vi "OEE_MAIN.vi"() -> ()   [LabVIEW 2020]
uses:
  OEE/FGV/SQL_raw_data/OEE_SQL_raw_data.ctl
  OEE/ini/typedef/OEE_all_config_info.ctl
  OEE/ini/typedef/OEE_main_ini_file.ctl
  OEE/queues/typedef/OEE_queue_refnums.ctl
  OEE/queues/typedef/OEE_MAIN_queue_element.ctl
  OEE/MAIN/OEE_MAIN_sequence_state.ctl
  OEE/queues/typedef/OEE_SCREEN_1_queue_element.ctl
  OEE/SCREEN_1/OEE_SCREEN_1_sequence_state.ctl
  OEE/queues/typedef/OEE_SCREEN_2_queue_element.ctl
  OEE/SCREEN_2/OEE_SCREEN_2_sequence_state.ctl
  OEE/queues/typedef/OEE_PULSE_queue_element.ctl
  OEE/PULSE/OEE_PULSE_sequence_state.ctl
  OEE/queues/typedef/OEE_GRAPH_TOGGLE_TIMER_queue_element.ctl
  OEE/SCREEN_2/GRAPH_TOGGLE_TIMER/OEE_GRAPH_TOGGLE_TIMER_sequence_state.ctl
  OEE/FGV/SQL_connection/FGV_OEE_SQL_connection.ctl
  OEE/FGV/SQL_raw_data/FGV_OEE_SQL_raw_data.ctl
  OEE/FGV/reference_selector/FGV_OEE_reference_selector.ctl
  OEE/FGV/reference_selector/OEE_reference_selecotr_references.ctl
  _misc/AULocalize/SubVIs/RegisterVI.vi
  _misc/AULocalize/SubVIs/Get Localized Phrase Compact Interface 0D.vi
panel:
  out "language_header":string caption="ЯЗЫК"
  out "status_info_header":string caption="ИНФОРМАЦИЯ О СТАТУСЕ"
  out "reference_selector_header":string caption="ТИП ДЕТАЛИ"
  out "time_source_header":string caption="TIME SOURCE"
  in  "language_russian":bool
  in  "language_english":bool
  in  "time_selector_btn":bool
  in  "time_selector":timestamp format="%<%x %H:%M:%S>T"
  in  "time_source_selector":enum32{"system_time", "manual_time"}(radio)
  in  "reload_reference_list":bool
  in  "reference_selector":u16(ring) items=["REF_1", "REF_2"]
  out "SQL_raw_data_out":T1
  out "update_pulse":bool=TRUE caption="Update Pulse:"
  in  "toggle_pulses":bool
  out "SQL_connection_status":bool=TRUE caption="SQL Connection Status:"
  in  "STOP":bool
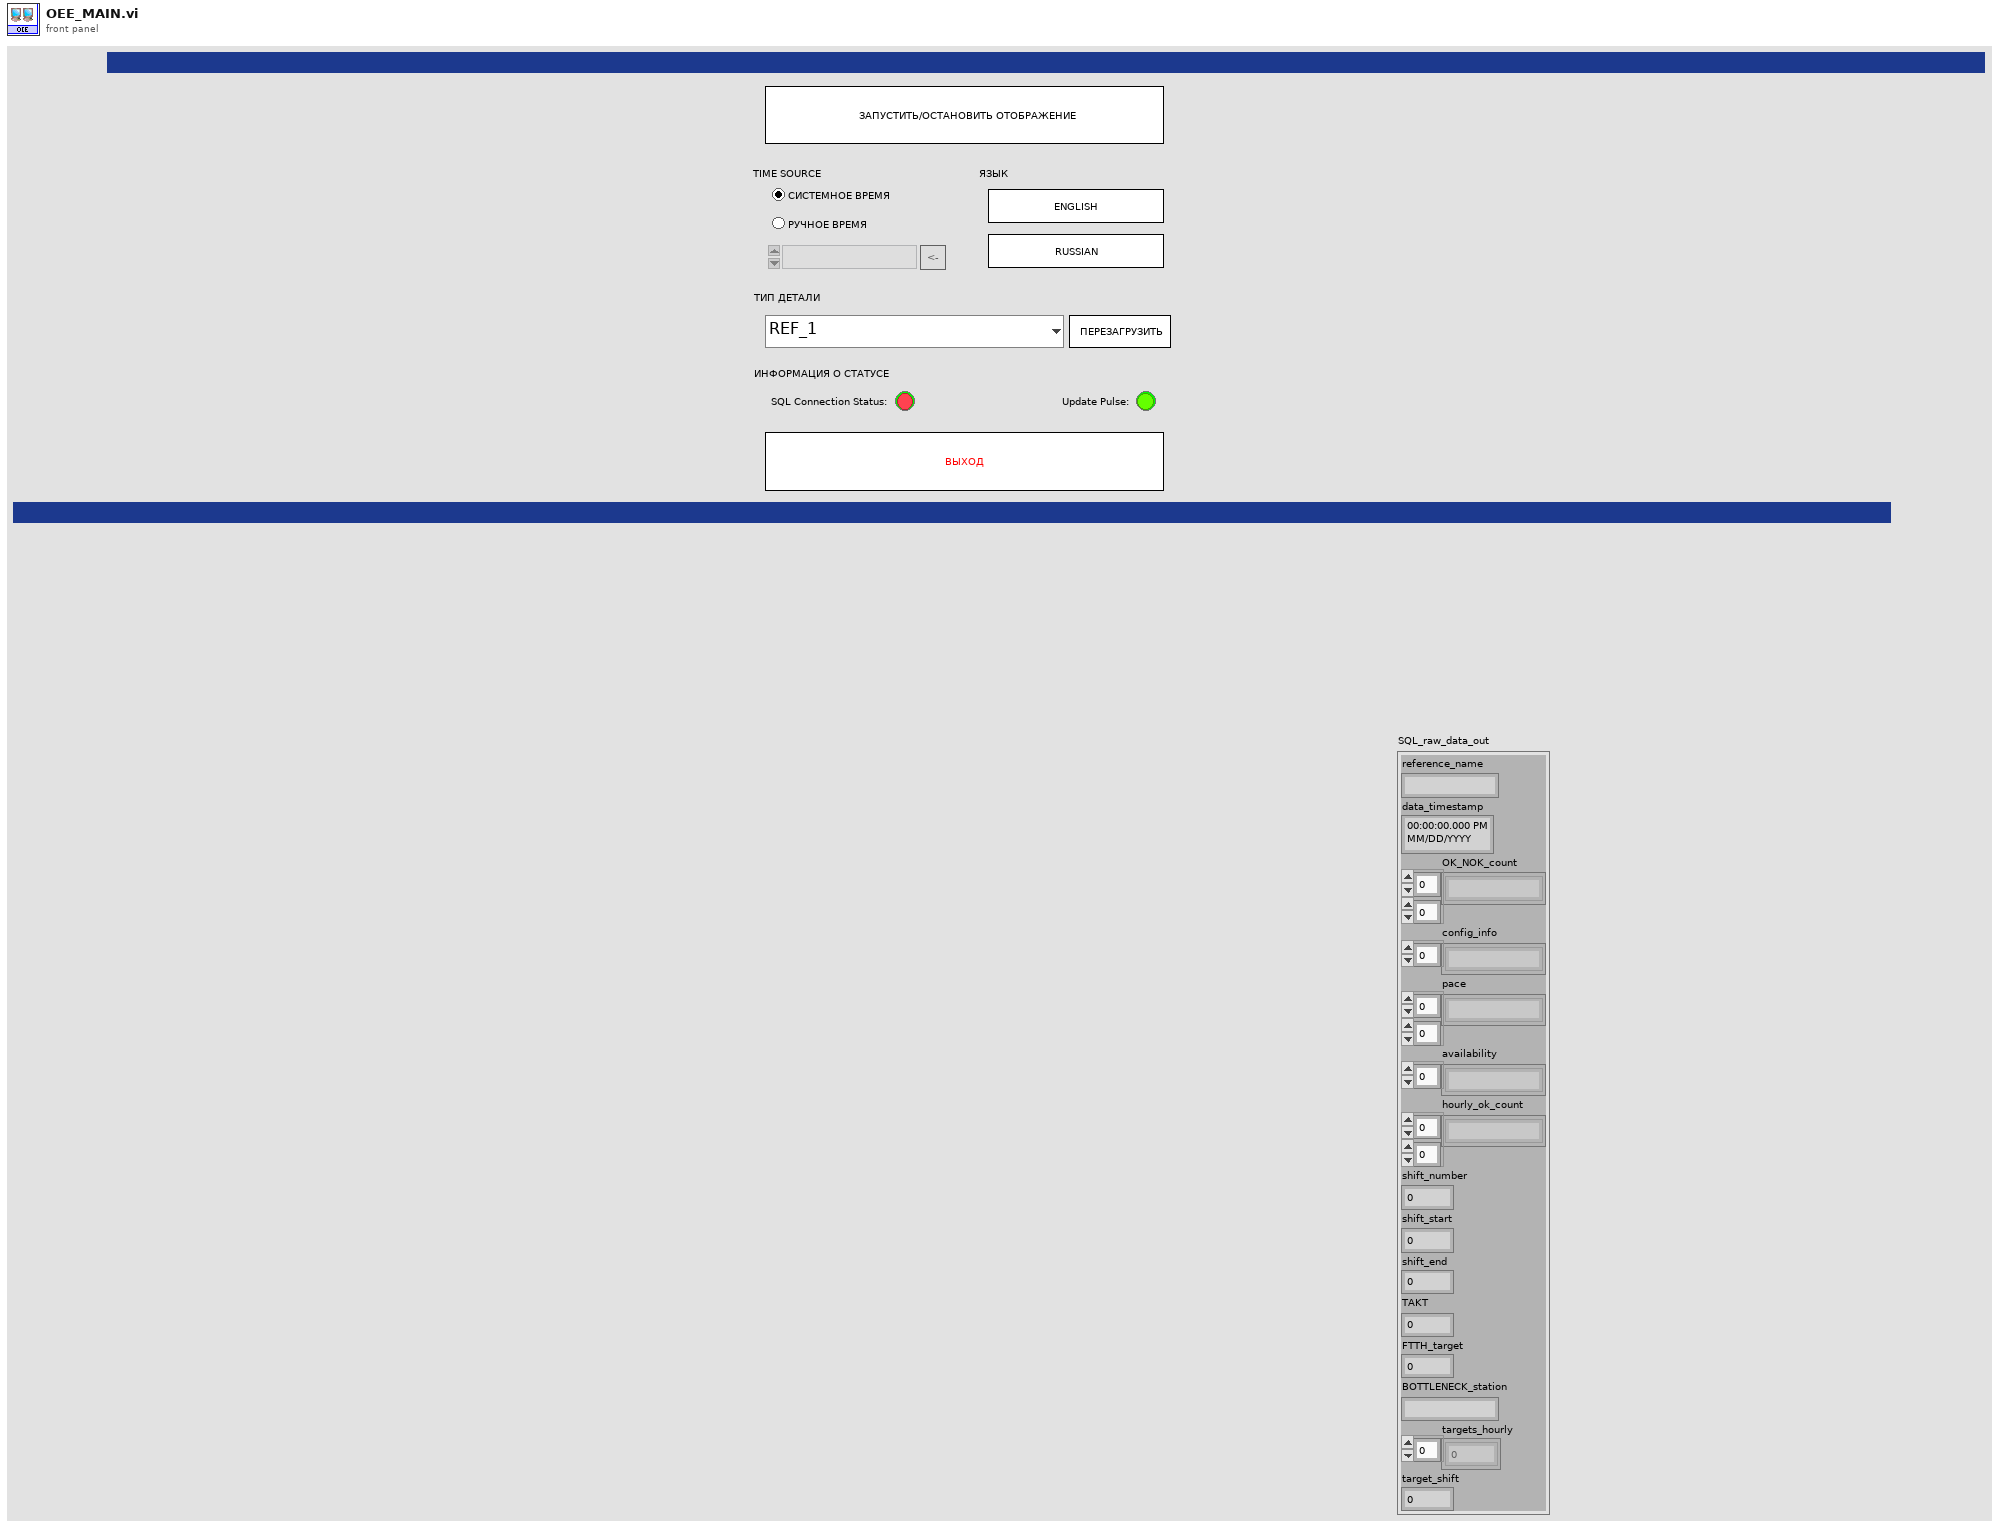
[diagram p1: front panel]
types:
  T1 = typedef "OEE_SQL_raw_data.ctl" = cluster{"reference_name":string, "data_timestamp":timestamp, "OK_NOK_count":string[][], "config_info":string[], "pace":string[][], "availability":string[], "hourly_ok_count":string[][], "shift_number":i8, "shift_start":i8, "shift_end":i8, "TAKT":u16, "FTTH_target":u16, "BOTTLENECK_station":string, "targets_hourly":u16[], "target_shift":u16}
  T2 = typedef "OEE_reference_selecotr_references.ctl" = cluster{"reference_list":string[], "reference_selector":refnum<vi>, "reload_reference_list":refnum<vi>, "toggle_pulses":refnum<vi>}
  T3 = typedef "FGV_OEE_reference_selector.ctl" = enum16{"initialize", "set_values", "enable", "disable", "disable_gray", "get_reference_list", "get_active_reference"}
  T4 = typedef "FGV_OEE_SQL_raw_data.ctl" = enum16{"initialize", "set_reference_name", "set_timestamp", "set_OK_NOK_count", "set_config_info", "set_pace", "set_availability", "set_hourly_ok_count", "set_targets", "get_all_info"}
  T5 = typedef "FGV_OEE_SQL_connection.ctl" = enum16{"initialize", "connect", "read_tables", "read_columns", "SELECT", "INSERT", "UPDATE", "DELETE", "EXEC + headers", "EXEC", "TRANSACTION", "connection_active?", "disconnect"}
  T6 = typedef "OEE_all_config_info.ctl" = cluster{"main_ini_file":T7, "SQL Password":string, "queue_refnums":T8}
  T7 = typedef "OEE_main_ini_file.ctl" = cluster{"SQL Driver":string, "SQL Server":string, "SQL Database":string, "SQL UID":string, "Reference table":string, "Reference history":string, "Archivisation CFG table":string, "Archivisation CFG history":string, "User table":string, "User history":string, "Default reference":string, "Update pulse[ms]":i32, "default language":string, "SCREEN 1 Left":i16, "SCREEN 1 Top":i16, "SCREEN 1 Width":i16, "SCREEN 1 Height":i16, "SCREEN 2 Left":i16, "SCREEN 2 Top":i16, "SCREEN 2 Width":i16, "SCREEN 2 Height":i16}
  T8 = typedef "OEE_queue_refnums.ctl" = cluster{"MAIN_queue":refnum<queue>, "SCREEN_1_queue":refnum<queue>, "SCREEN_2_queue":refnum<queue>, "PULSE_queue":refnum<queue>, "GRAPH_TOGGLE_queue":refnum<queue>}
  T9 = typedef "OEE_MAIN_sequence_state.ctl" = enum16{"initialize", "get_next_state", "get_SQL_data", "update_displays", "error", "stop"}
  T10 = typedef "OEE_PULSE_sequence_state.ctl" = enum16{"initialize", "get_next_state", "start_pulses", "stop_pulses", "pulse", "error", "stop"}
  T11 = typedef "OEE_GRAPH_TOGGLE_TIMER_queue_element.ctl" = cluster{"state":T12, "variable":variant}
  T12 = typedef "OEE_GRAPH_TOGGLE_TIMER_sequence_state.ctl" = enum16{"initialize", "get_next_state", "start_toggling", "stop_toggling", "do_toggle", "error", "stop"}
  T13 = typedef "OEE_PULSE_queue_element.ctl" = cluster{"state":T10, "variable":variant}
  T14 = typedef "OEE_MAIN_queue_element.ctl" = cluster{"state":T9, "variable":variant}
  T15 = typedef "OEE_SCREEN_1_queue_element.ctl" = cluster{"state":T16, "variable":variant}
  T16 = typedef "OEE_SCREEN_1_sequence_state.ctl" = enum16{"initialize", "get_next_state", "update", "show", "hide", "error", "stop"}
  T17 = typedef "OEE_SCREEN_2_queue_element.ctl" = cluster{"state":T18, "variable":variant}
  T18 = typedef "OEE_SCREEN_2_sequence_state.ctl" = enum16{"initialize", "get_next_state", "update", "show", "hide", "error", "stop"}
  T19 = enum8{"Enabled", "Disabled", "Disabled and Grayed Out"}
  T20 = typedef "SCREEN_1.ctl" = cluster{"header_date":string, "header_time":string, "header_takt":string, "header_shift":string, "OP10_actual":string, "OP10_rejects":string, "OP10_quality_yeild":string, "OP10_pace":string, "OP20_actual":string, "OP20_rejects":string, "OP20_quality_yeild":string, "OP20_pace":string, "OP30_actual":string, "OP30_rejects":string, "OP30_quality_yeild":string, "OP30_pace":string, "OP40_actual":string, "OP40_rejects":string, "OP40_quality_yeild":string, "OP40_pace":string, "OP50_actual":string, "OP50_rejects":string, "OP50_quality_yeild":string, "OP50_pace":string, "OP60_actual":string, "OP60_rejects":string, "OP60_quality_yeild":string, "OP60_pace":string, "OP70_actual":string, "OP70_rejects":string, "OP70_quality_yeild":string, "OP70_pace":string, "OP80_actual":string, "OP80_rejects":string, "OP80_quality_yeild":string, "OP80_pace":string, "OP90_actual":string, "OP90_rejects":string, "OP90_quality_yeild":string, "OP90_pace":string, "OP100_actual":string, "OP100_rejects":string, "OP100_quality_yeild":string, "OP100_pace":string, "OP110_actual":string, "OP110_rejects":string, "OP110_quality_yeild":string, "OP110_pace":string, "OP120_actual":string, "OP120_rejects":string, "OP120_quality_yeild":string, "OP120_pace":string, "OP130_actual":string, "OP130_rejects":string, "OP130_quality_yeild":string, "OP130_pace":string, "OP10_header":string, "OP20_header":string, "OP30_header":string, "OP40_header":string, "OP50_header":string, "OP60_header":string, "OP70_header":string, "OP80_header":string, "OP90_header":string, "OP100_header":string, "OP110_header":string, "OP120_header":string, "OP130_header":string, "additional_info":string, "bottleneck_OP":string, "bottleneck_header":string, "screen_1_header":string, "actual_header":string, "rejects_header":string, "FTTH_header":string, "pace_header":string, "actual_header":string, "rejects_header":string, "FTTH_header":string, "pace_header":string}
  T21 = typedef "SCREEN_2.ctl" = cluster{"header_part_no":string, "header_customer":string, "performance_percentage":string, "performance_target":string, "performance_actual":string, "performance_header":string, "performance_target_header":string, "performance_actual_header":string, "screen_2_header":string}
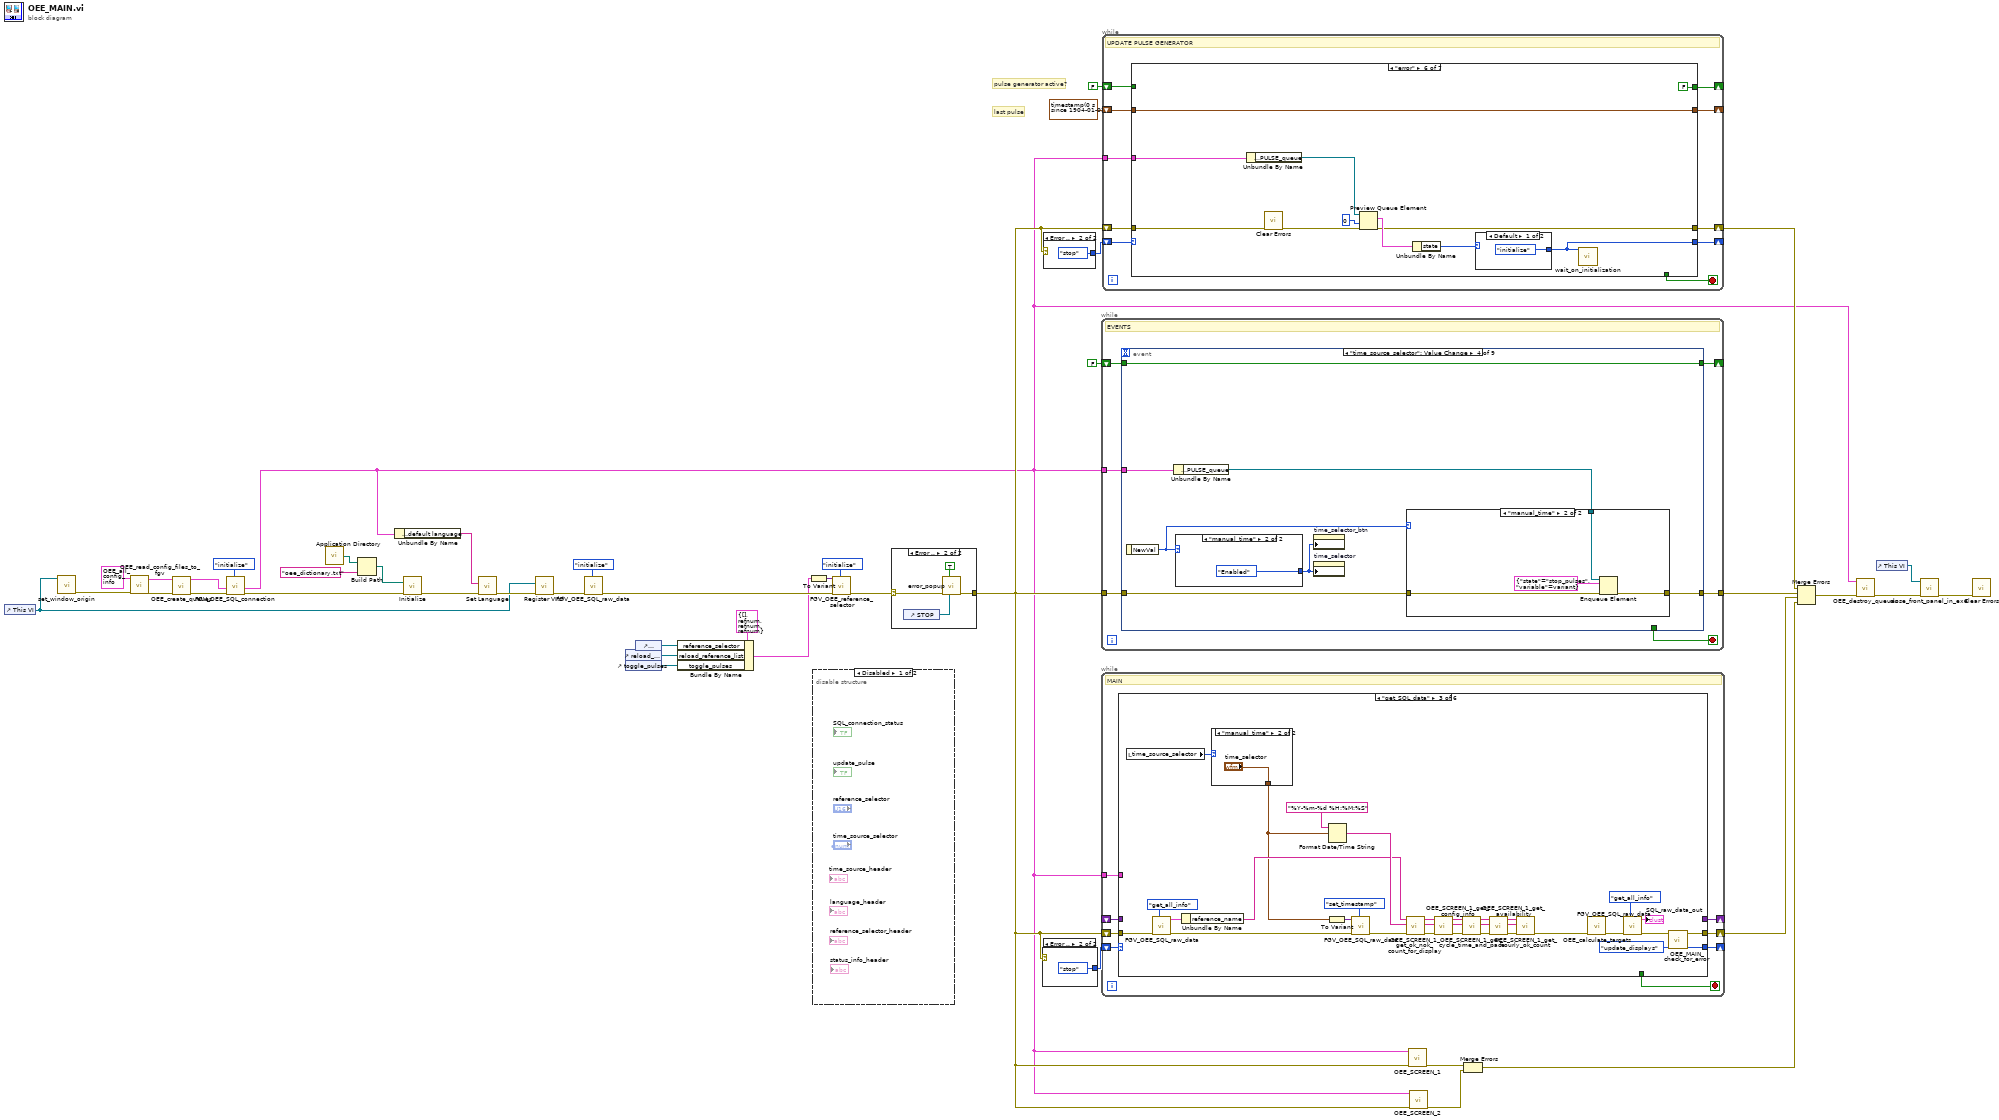
[diagram p0: block diagram]
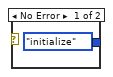
[diagram p2: hidden frame]
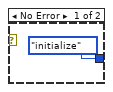
[diagram p3: hidden frame]
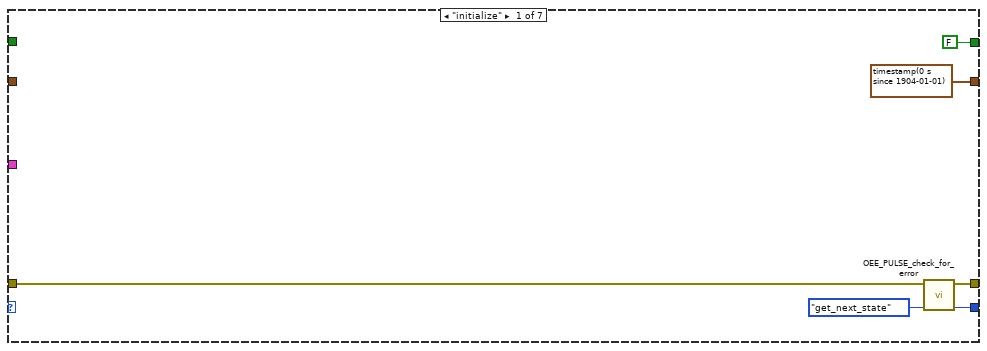
[diagram p5: hidden frame]
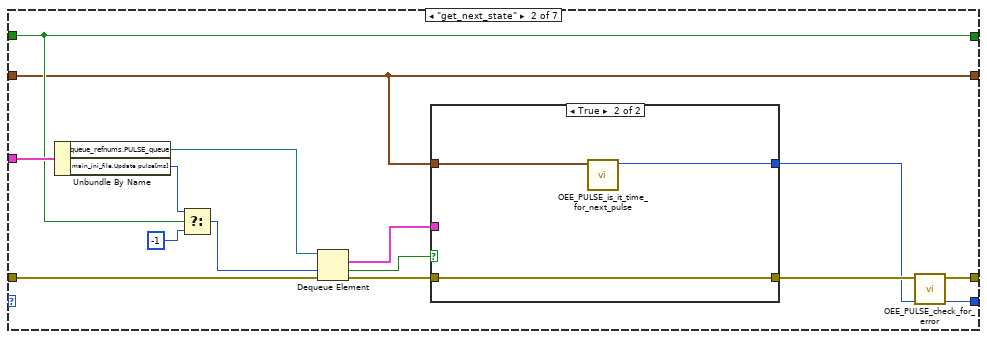
[diagram p6: hidden frame]
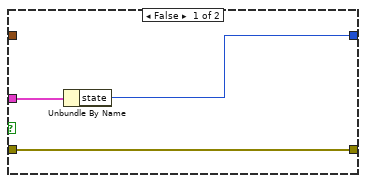
[diagram p7: hidden frame]
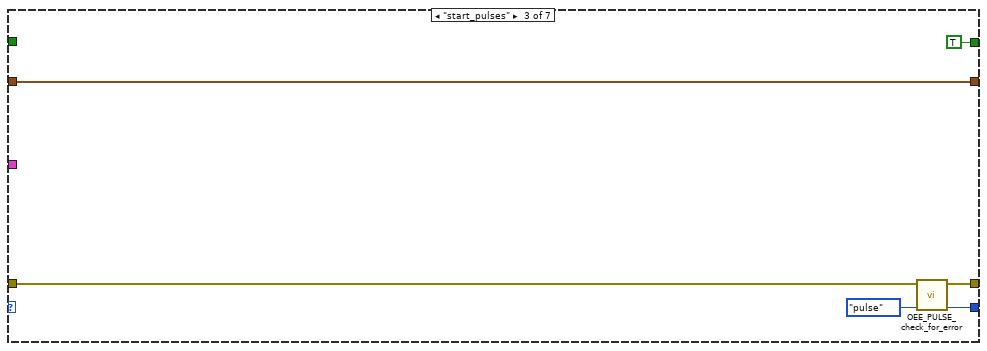
[diagram p8: hidden frame]
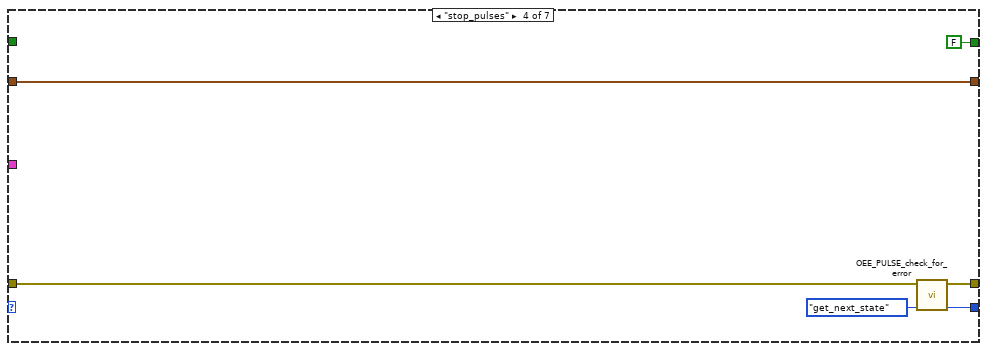
[diagram p9: hidden frame]
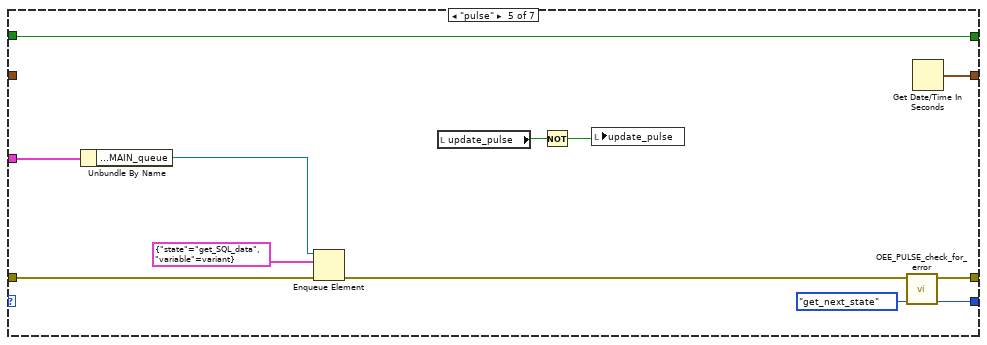
[diagram p10: hidden frame]
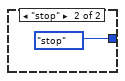
[diagram p11: hidden frame]
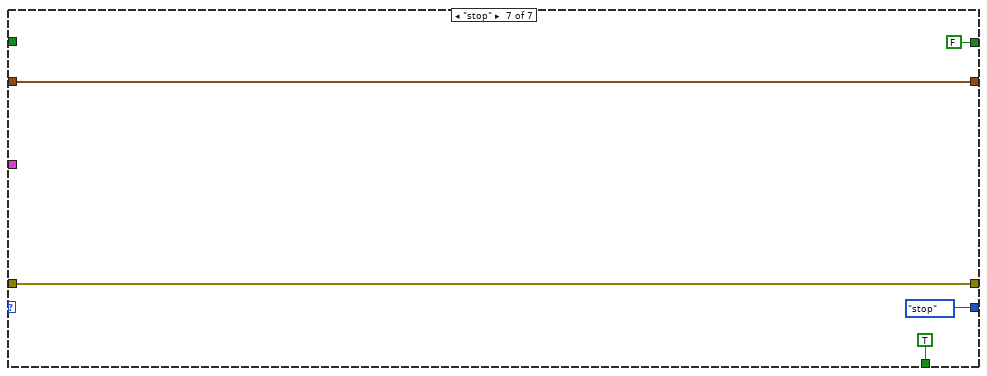
[diagram p12: hidden frame]
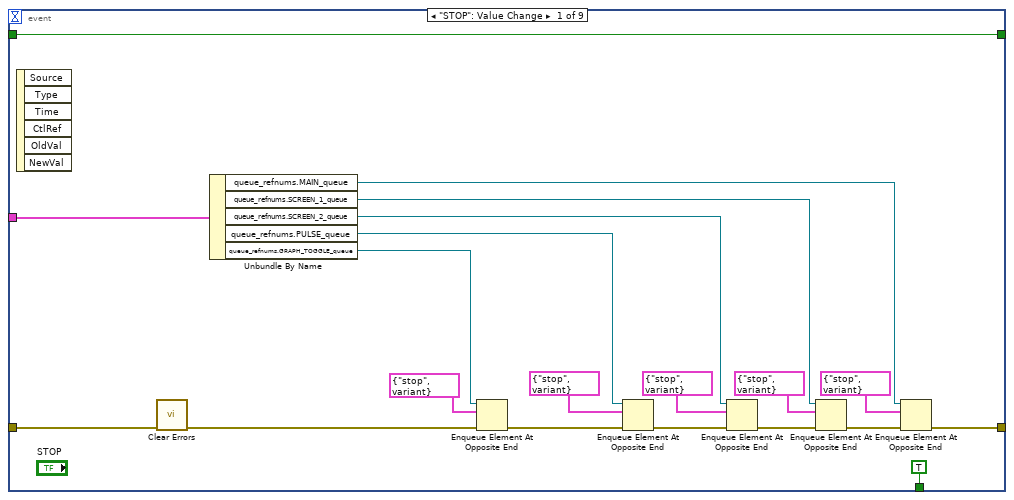
[diagram p14: hidden frame]
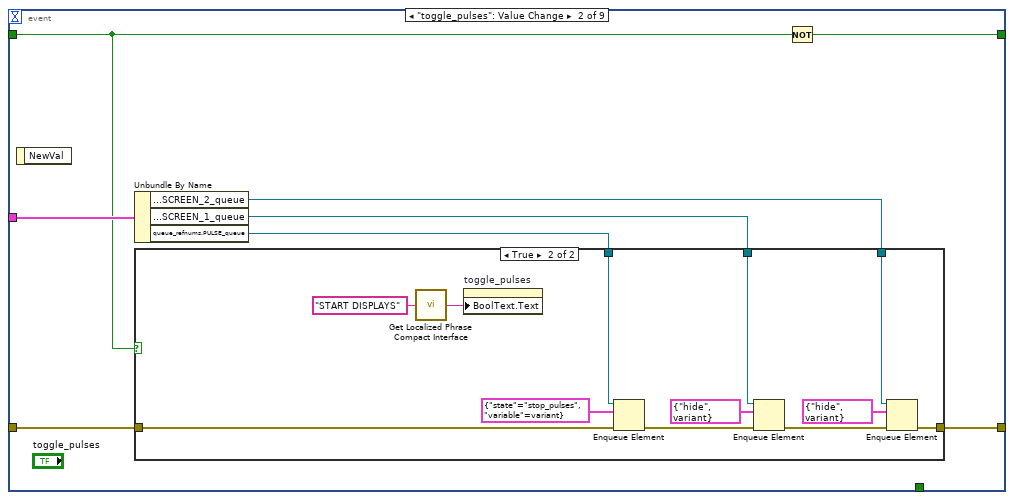
[diagram p15: hidden frame]
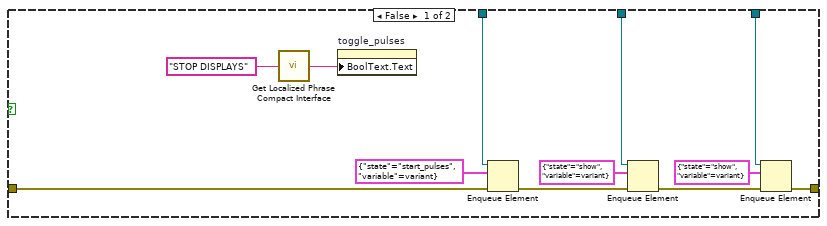
[diagram p16: hidden frame]
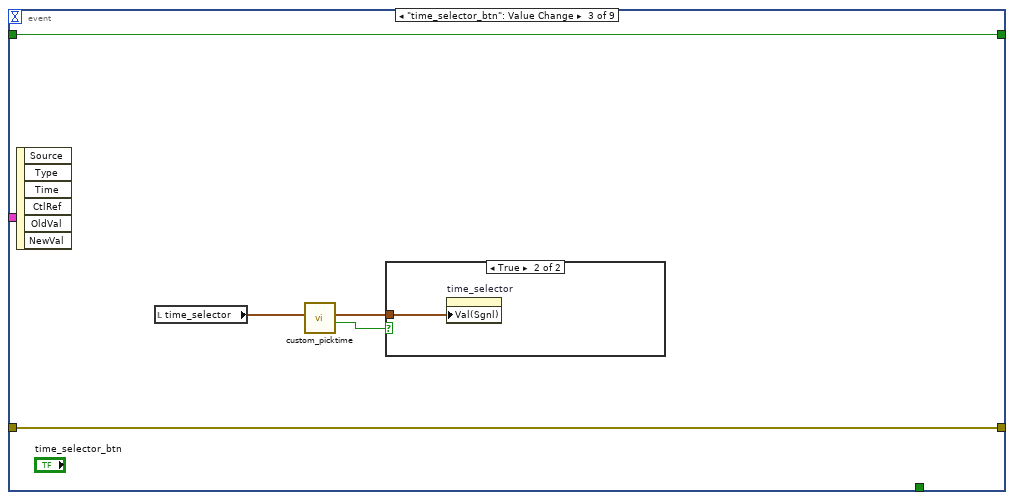
[diagram p17: hidden frame]
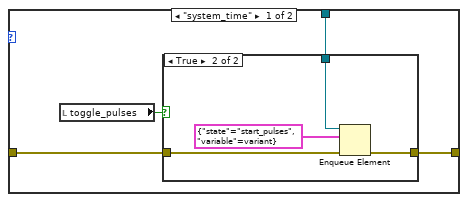
[diagram p19: hidden frame]
diagram:
  # "last pulse"
  # "pulse generator active?"
  n1 = control-ref of="This VI"() -> (w2:refnum<vi>)
  n2 = call "set_window_origin.vi"("this_vi_reference"=w2) -> ("error_out"=w38:errorcluster)  [unwired: 10 in]
  n3 = call "OEE_read_config_files_to_fgv.vi"("error_in"=w38, "all_config_info_in"=T6 {"main_ini_file"={"SQL Driver"="", "SQL Server"="", "SQL Database"="", "SQL UID"="", "Reference table"="", "Reference history"="", "Archivisation CFG table"="", "Archivisation CFG history"="", "User table"="", "User history"="", "Default reference"="", "Update pulse[ms]"=0, "default language"="", "SCREEN 1 Left"=0, "SCREEN 1 Top"=0, "SCREEN 1 Width"=0, "SCREEN 1 Height"=0, "SCREEN 2 Left"=0, "SCREEN 2 Top"=0, "SCREEN 2 Width"=0, "SCREEN 2 Height"=0}, "SQL Password"="", "queue_refnums"={"MAIN_queue"=refnum, "SCREEN_1_queue"=refnum, "SCREEN_2_queue"=refnum, "PULSE_queue"=refnum, "GRAPH_TOGGLE_queue"=refnum}} ("all_config_info")) -> ("error_out"=w41:errorcluster, "all_config_info_out"=w42:T6)  [unwired: 8 in]
  n4 = call "OEE_create_queues.vi"("error_in"=w41, "all_config_info_in"=w42) -> ("error_out"=w32:errorcluster, "all_config_info_out"=w31:T6)  [unwired: 8 in]
  n5 = call "FGV_OEE_SQL_connection.vi"("options"=FGV_OEE_SQL_connection."initialize", "error_in"=w32, "all_config_info_in"=w31) -> ("error_out"=w3:errorcluster, "all_config_info_out"=w1:T6)  [unwired: 4 in, 3 out]
  n6 = call <vilib>:"Application Directory.vi"() -> ("Application Directory"=w10:path)
  n7 = Build Path(base path=w10, name or relative path="oee_dictionary.txt") -> (appended path=w8:path)
  n8 = Unbundle By Name(w1) -> ("main_ini_file.default language"=w5:string)
  n9 = call "Initialize.vi"("Dictionary File Path"=w8, "error in"=w3) -> ("error out"=w7:errorcluster)  [unwired: 8 in, 5 out]
  n10 = call "Set Language.vi"("error in"=w7, "Target Language (current lang)"=w5) -> ("error out"=w6:errorcluster)  [unwired: 8 in, 1 out]
  n11 = call-poly "Register VI(s).vi"("error in"=w6, "VI Ref"=w2) -> ("error out"=w4:errorcluster)  [unwired: 8 in, 1 out]
  n12 = call "FGV_OEE_SQL_raw_data.vi"("options"=FGV_OEE_SQL_raw_data."initialize", "error_in"=w4) -> ("error_out"=w21:errorcluster)  [unwired: 8 in, 1 out]
  n13 = control-ref of="reload_reference_list"() -> (w16:refnum<vi>)
  n14 = control-ref of="toggle_pulses"() -> (w15:refnum<vi>)
  n15 = control-ref of="reference_selector"() -> (w17:refnum<vi>)
  n16 = Bundle By Name(cluster=T2 {"reference_list"=[], "reference_selector"=refnum, "reload_reference_list"=refnum, "toggle_pulses"=refnum} ("OBJ_references"), "reference_selector"=w17, "reload_reference_list"=w16, "toggle_pulses"=w15) -> (w13:T2)
  n17 = To Variant(anything=w13) -> (Variant=w14:variant)
  n18 = disable-structure shown="Disabled" {
    frame Disabled {
    }
    frame Enabled {
    }
  }
  n19 = call "FGV_OEE_reference_selector.vi"("options"=FGV_OEE_reference_selector."initialize", "error_in"=w21, "input"=w14) -> ("error_out"=w12:errorcluster)  [unwired: 7 in, 1 out]
  n20 = case shown="Error .." w12 {
    selector: w12 -> [w44 w47]
    tunnel: [w44 w48] -> w11
    frame No Error {
    }
    frame Error {
      n21 = control-ref of="STOP"() -> (w45:refnum<vi>)
      n22 = call "error_popup.vi"("STOP_button_reference"=w45, "EXIT App If Error? (F)"=TRUE, "error_in"=w47) -> ("error_out"=w48:errorcluster)  [unwired: 8 in]
    }
  }
  n23 = case shown="Error .." w11 {
    tunnel: [OEE_MAIN_sequence_state."initialize" ("OEE_MAIN_sequence_state") OEE_MAIN_sequence_state."stop" ("OEE_MAIN_sequence_state")] -> w33
    frame No Error {
    }
    frame Error {
    }
  }
  n24 = case shown="Error .." w11 {
    tunnel: [OEE_PULSE_sequence_state."initialize" ("GUI_TIMER_loop_state_in") OEE_PULSE_sequence_state."stop" ("GUI_TIMER_loop_state_in")] -> w25
    frame No Error {
    }
    frame Error {
    }
  }
  n25 = while {
    tunnel: w11 -> [w56]
    tunnel: [w58] -> w37
    tunnel: w1 -> [w55]
    shift-right: [w54] -> _
    shift-left: FALSE ("NewVal") -> [w53]
    stop <- w57 stop-if-true
    # "EVENTS"
    n26 = event shown="[3] \"time_source_selector\": Value Change" {
      selector: _ -> [_ _ _ _ _ _ _ _ _]
      dyn-events: _ -> [_ _ _ _ _ _ _ _ _]
      timeout: _ -> [_ _ _ _ _ _ _ _ _]
      tunnel: w56 -> [w76 w85 w114 w122 w142 w153 w163 w169 w172]
      tunnel: [w70 w84 w114 w121 w141 w145 w161 w169 w172] -> w58
      tunnel: [TRUE _ _ _ _ _ _ _ _] -> w57
      tunnel: w55 -> [w77 w86 _ w120 w143 w146 _ _ _]
      tunnel: [w59 w82 w115 w123 w144 w159 w160 w170 w173] -> w54
      tunnel: w53 -> [w59 w81 w115 w123 w144 w159 w160 w170 w173]
      event "STOP": Value Change {
        n27 = event-data() -> ()  [unwired: 1 in, 6 out]
        n28 = call <vilib>:"Clear Errors.vi"("error in (no error)"=w76) -> ("error out"=w63:errorcluster)  [unwired: 5 in, 1 out]
        n29 = Unbundle By Name(w77) -> ("queue_refnums.MAIN_queue"=w75:refnum<queue>, "queue_refnums.SCREEN_1_queue"=w73:refnum<queue>, "queue_refnums.SCREEN_2_queue"=w71:refnum<queue>, "queue_refnums.PULSE_queue"=w65:refnum<queue>, "queue_refnums.GRAPH_TOGGLE_queue"=w61:refnum<queue>)
        n30 = Enqueue Element At Opposite End(queue=w61, element=T11 {"state"=enum."stop", "variable"=variant}, error in (no error)=w63) -> (error out=w62:errorcluster)  [unwired: 1 in, 2 out]
        n31 = Enqueue Element At Opposite End(queue=w65, element=T13 {"state"=enum."stop", "variable"=variant}, error in (no error)=w62) -> (error out=w66:errorcluster)  [unwired: 1 in, 2 out]
        n32 = Enqueue Element At Opposite End(queue=w71, element=T17 {"state"=enum."stop", "variable"=variant}, error in (no error)=w66) -> (error out=w72:errorcluster)  [unwired: 1 in, 2 out]
        n33 = Enqueue Element At Opposite End(queue=w73, element=T15 {"state"=enum."stop", "variable"=variant}, error in (no error)=w72) -> (error out=w74:errorcluster)  [unwired: 1 in, 2 out]
        n34 = Enqueue Element At Opposite End(queue=w75, element=T14 {"state"=enum."stop", "variable"=variant}, error in (no error)=w74) -> (error out=w70:errorcluster)  [unwired: 1 in, 2 out]
      }
      event "toggle_pulses": Value Change {
        n35 = event-data() -> ()  [unwired: 1 in, 1 out]
        n36 = Unbundle By Name(w86) -> ("queue_refnums.SCREEN_2_queue"=w79:refnum<queue>, "queue_refnums.SCREEN_1_queue"=w80:refnum<queue>, "queue_refnums.PULSE_queue"=w83:refnum<queue>)
        n37 = case shown="True" w81 {
          tunnel: w85 -> [w88 w104]
          tunnel: [w89 w102] -> w84
          tunnel: w83 -> [w98 w110]
          tunnel: w80 -> [w94 w106]
          tunnel: w79 -> [w91 w101]
          frame False {
            n38 = call-poly "Get Localized Phrase Compact Interface.vi"("Key"="STOP DISPLAYS" ("Boolean Text.Text")) -> ("Translated Phrase"=w87:string)
            n39 = property on="toggle_pulses" class="Bool (strict)"("BoolText.Text"=w87) -> ()  [unwired: 2 in, 2 out]
            n40 = Enqueue Element(queue=w98, element=T13 {"state"=enum."start_pulses", "variable"=variant}, error in (no error)=w88) -> (error out=w95:errorcluster)  [unwired: 1 in, 2 out]
            n41 = Enqueue Element(queue=w94, element=T15 {"state"=enum."show", "variable"=variant}, error in (no error)=w95) -> (error out=w90:errorcluster)  [unwired: 1 in, 2 out]
            n42 = Enqueue Element(queue=w91, element=T17 {"state"=enum."show", "variable"=variant}, error in (no error)=w90) -> (error out=w89:errorcluster)  [unwired: 1 in, 2 out]
          }
          frame True {
            n43 = call-poly "Get Localized Phrase Compact Interface.vi"("Key"="START DISPLAYS" ("Boolean Text.Text")) -> ("Translated Phrase"=w99:string)
            n44 = property on="toggle_pulses" class="Bool (strict)"("BoolText.Text"=w99) -> ()  [unwired: 2 in, 2 out]
            n45 = Enqueue Element(queue=w110, element=T13 {"state"=enum."stop_pulses", "variable"=variant}, error in (no error)=w104) -> (error out=w107:errorcluster)  [unwired: 1 in, 2 out]
            n46 = Enqueue Element(queue=w106, element=T15 {"state"=enum."hide", "variable"=variant}, error in (no error)=w107) -> (error out=w103:errorcluster)  [unwired: 1 in, 2 out]
            n47 = Enqueue Element(queue=w101, element=T17 {"state"=enum."hide", "variable"=variant}, error in (no error)=w103) -> (error out=w102:errorcluster)  [unwired: 1 in, 2 out]
          }
        }
        n48 = Not(x=w81) -> (.not. x?=w82:bool)
      }
      event "time_selector_btn": Value Change {
        n49 = event-data() -> ()  [unwired: 1 in, 6 out]
        n50 = local read "time_selector"() -> (w113:timestamp)
        n51 = call "custom_picktime.vi"("secin"=w113) -> ("ok"=w112:bool, "secout"=w111:timestamp)  [unwired: 9 in]
        n52 = case shown="True" w112 {
          tunnel: w111 -> [_ w116]
          frame False {
          }
          frame True {
            n53 = property on="time_selector" class="AbsTime (strict)"("Val(Sgnl)"=w116) -> ()  [unwired: 2 in, 2 out]
          }
        }
      }
      event "time_source_selector": Value Change {
        n54 = event-data() -> ("NewVal"=w118:enum32{"system_time", "manual_time"})  [unwired: 1 in]
        n55 = Unbundle By Name(w120) -> ("queue_refnums.PULSE_queue"=w119:refnum<queue>)
        n56 = case shown="\"manual_time\"" w118 {
          tunnel: [T19."Disabled and Grayed Out" ("Disabled") T19."Enabled" ("Disabled")] -> w117
          frame "system_time" {
          }
          frame "manual_time" {
          }
        }
        n57 = property on="time_selector_btn" class="Bool"("DisabledEnum"=w117) -> ()  [unwired: 2 in, 2 out]
        n58 = property on="time_selector" class="AbsTime (strict)"("DisabledEnum"=w117) -> ()  [unwired: 2 in, 2 out]
        n59 = case shown="\"manual_time\"" w118 {
          tunnel: w122 -> [w127 w136]
          tunnel: [w126 w135] -> w121
          tunnel: w119 -> [w125 w134]
          frame "system_time" {
            n60 = local read "toggle_pulses"() -> (w124:bool)
            n61 = case shown="True" w124 {
              tunnel: w127 -> [w128 w132]
              tunnel: [w128 w131] -> w126
              tunnel: w125 -> [_ w130]
              frame False {
              }
              frame True {
                n62 = Enqueue Element(queue=w130, element=T13 {"state"=enum."start_pulses", "variable"=variant}, error in (no error)=w132) -> (error out=w131:errorcluster)  [unwired: 1 in, 2 out]
              }
            }
          }
          frame "manual_time" {
            n63 = Enqueue Element(queue=w134, element=T13 {"state"=enum."stop_pulses", "variable"=variant}, error in (no error)=w136) -> (error out=w135:errorcluster)  [unwired: 1 in, 2 out]
          }
        }
      }
      event "time_selector": Value Change {
        n64 = event-data() -> ()  [unwired: 1 in, 1 out]
        n65 = Unbundle By Name(w143) -> ("queue_refnums.MAIN_queue"=w140:refnum<queue>)
        n66 = Enqueue Element(queue=w140, element=T14 {"state"=enum."get_SQL_data", "variable"=variant}, error in (no error)=w142) -> (error out=w141:errorcluster)  [unwired: 1 in, 2 out]
      }
      event "reference_selector": Value Change {
        n67 = event-data() -> ()  [unwired: 1 in, 1 out]
        n68 = call "FGV_OEE_reference_selector.vi"("options"=FGV_OEE_reference_selector."get_active_reference", "error_in"=w153) -> ("error_out"=w152:errorcluster, "output"=w156:variant)  [unwired: 8 in]
        n69 = Variant To Data(error in=w152, type="", Variant=w156) -> (data=w158:string, error out=w151:errorcluster)
        n70 = To Variant(anything=w158) -> (Variant=w157:variant)
        n71 = call "FGV_OEE_SQL_raw_data.vi"("options"=FGV_OEE_SQL_raw_data."set_reference_name", "error_in"=w151, "input"=w157) -> ("error_out"=w147:errorcluster)  [unwired: 7 in, 1 out]
        n72 = Unbundle By Name(w146) -> ("queue_refnums.MAIN_queue"=w149:refnum<queue>)
        n73 = Enqueue Element(queue=w149, element=T14 {"state"=enum."get_SQL_data", "variable"=variant}, error in (no error)=w147) -> (error out=w145:errorcluster)  [unwired: 1 in, 2 out]
      }
      event "reload_reference_list": Value Change {
        n74 = event-data() -> ()  [unwired: 1 in, 6 out]
        n75 = call "FGV_OEE_SQL_connection.vi"("options"=FGV_OEE_SQL_connection."EXEC", "error_in"=w163, "SQL_statement"="EXEC OEEGetReferenceList") -> ("error_out"=w162:errorcluster, "SQL_result"=w164:variant)  [unwired: 4 in, 3 out]
        n76 = call "FGV_OEE_reference_selector.vi"("options"=FGV_OEE_reference_selector."set_values", "error_in"=w162, "input"=w164) -> ("error_out"=w161:errorcluster)  [unwired: 7 in, 1 out]
      }
      event "language_english": Value Change {
        n77 = event-data() -> ()  [unwired: 1 in, 6 out]
        n78 = call "Set Language.vi"("Target Language (current lang)"="English") -> ()  [unwired: 9 in, 2 out]
      }
      event "language_russian": Value Change {
        n79 = event-data() -> ()  [unwired: 1 in, 6 out]
        n80 = call "Set Language.vi"("Target Language (current lang)"="Russian") -> ()  [unwired: 9 in, 2 out]
      }
    }
  }
  n81 = while {
    tunnel: w1 -> [w177]
    shift-right: [w178] -> _
    shift-left: w33 -> [w179]
    shift-right: [w176] -> _
    shift-left: _ -> [w175]
    shift-right: [w180] -> w36
    shift-left: w11 -> [w181]
    stop <- w174 stop-if-true
    # "MAIN"
    n82 = case shown="\"get_SQL_data\"" w179 {
      tunnel: w181 -> [w201 w210 w223 w265 w269 w294]
      tunnel: [w204 w214 w246 w268 w272 w294] -> w180
      tunnel: [w202 w213 w245 w267 w271 OEE_MAIN_sequence_state."stop" ("OEE_MAIN_sequence_state")] -> w178
      tunnel: w177 -> [w184 w208 _ w262 w270 _]
      tunnel: [_ w206 _ _ _ _] -> w176
      tunnel: w175 -> [_ _ _ _ _ _]
      tunnel: [_ _ _ _ _ TRUE] -> w174
      frame "initialize" {
        # "timer to wait on screen vi's initialization\nif any problems with missing references in fgv occur or something,\ndo proper initialization with waiting for ready message from threads"
        n83 = call "FGV_OEE_SQL_connection.vi"("options"=FGV_OEE_SQL_connection."connect", "error_in"=w201) -> ("error_out"=w196:errorcluster)  [unwired: 5 in, 4 out]
        n84 = Unbundle By Name(w196) -> ("status"=w199:bool)
        n85 = call-poly "Get Localized Phrase Compact Interface.vi"("Key"="START DISPLAYS" ("Boolean Text.Text")) -> ("Translated Phrase"=w182:string)
        n86 = local write "STOP"(FALSE ("STOP")) -> ()
        n87 = Get Date/Time In Seconds() -> (seconds since 1Jan1904=w189:timestamp)
        n88 = property on="toggle_pulses" class="Bool (strict)"("BoolText.Text"=w182) -> ()  [unwired: 2 in, 2 out]
        n89 = local write "time_selector"(w189) -> ()
        n90 = local write "SQL_connection_status"(w199) -> ()
        n91 = property on="time_source_selector" class="RadioBtnsControl (strict)"("Val(Sgnl)"=enum32{"system_time", "manual_time"}."system_time" ("time_source_selector")) -> ()  [unwired: 2 in, 2 out]
        n92 = call "FGV_OEE_SQL_connection.vi"("options"=FGV_OEE_SQL_connection."EXEC", "error_in"=w196, "SQL_statement"="EXEC OEEGetReferenceList") -> ("error_out"=w193:errorcluster, "SQL_result"=w192:variant)  [unwired: 4 in, 3 out]
        n93 = call "FGV_OEE_reference_selector.vi"("options"=FGV_OEE_reference_selector."set_values", "error_in"=w193, "input"=w192) -> ("error_out"=w187:errorcluster)  [unwired: 7 in, 1 out]
        n94 = control-ref of="reference_selector"() -> (w185:refnum<vi>)
        n95 = call "OEE_MAIN_set_default_reference.vi"("all_config_info"=w184, "error_in"=w187, "reference_selector"=w185) -> ("error_out"=w186:errorcluster, "Default reference ok?"=w183:bool)  [unwired: 7 in]
        n96 = Wait (ms)(milliseconds to wait=u32 2000) -> ()  [unwired: 1 out]
        n97 = case shown="True" w183 {
          frame False {
          }
          frame True {
            n98 = property on="toggle_pulses" class="Bool (strict)"("Val(Sgnl)"=TRUE ("Value (Signaling)")) -> ()  [unwired: 2 in, 2 out]
          }
        }
        n99 = call "OEE_MAIN_check_for_error.vi"("MAIN_loop_state_in"=OEE_MAIN_sequence_state."get_next_state", "error_in"=w186) -> ("MAIN_loop_state_out"=w202:T9, "error_out"=w204:errorcluster)  [unwired: 8 in]
      }
      frame "get_next_state" {
        n100 = Unbundle By Name(w208) -> ("queue_refnums.MAIN_queue"=w211:refnum<queue>)
        n101 = Dequeue Element(queue=w211, error in (no error)=w210) -> (element=w212:T14, error out=w209:errorcluster)  [unwired: 1 in, 2 out]
        n102 = Unbundle By Name(w212) -> ("variable"=w206:variant, "state"=w207:T9)
        n103 = call "OEE_MAIN_check_for_error.vi"("MAIN_loop_state_in"=w207, "error_in"=w209) -> ("MAIN_loop_state_out"=w213:T9, "error_out"=w214:errorcluster)  [unwired: 8 in]
      }
      frame "get_SQL_data" {
        n104 = local read "time_source_selector"() -> (w219:enum32{"system_time", "manual_time"})
        n105 = call "FGV_OEE_SQL_raw_data.vi"("options"=FGV_OEE_SQL_raw_data."get_all_info", "error_in"=w223) -> ("error_out"=w222:errorcluster, "SQL_raw_data_out"=w221:T1)  [unwired: 8 in]
        n106 = Unbundle By Name(w221) -> ("reference_name"=w220:string)
        n107 = case shown="\"manual_time\"" w219 {
          tunnel: [w247 "time_selector"] -> w218
          frame "system_time" {
            n108 = Get Date/Time In Seconds() -> (seconds since 1Jan1904=w247:timestamp)
          }
          frame "manual_time" {
          }
        }
        n109 = To Variant(anything=w218) -> (Variant=w240:variant)
        n110 = Format Date/Time String(time format string (%c)="%Y-%m-%d %H:%M:%S", seconds (now)=w218) -> (date/time string=w227:string)  [unwired: 1 in]
        n111 = call "FGV_OEE_SQL_raw_data.vi"("options"=FGV_OEE_SQL_raw_data."set_timestamp", "error_in"=w222, "input"=w240) -> ("error_out"=w242:errorcluster)  [unwired: 7 in, 1 out]
        n112 = call "OEE_SCREEN_1_get_ok_nok_count_for_display.vi"("error_in"=w242, "current_time_in"=w227, "reference_name_in"=w220) -> ("error_out"=w239:errorcluster, "current_time_out"=w237:string, "reference_name_out"=w238:string)  [unwired: 6 in]
        n113 = call "OEE_SCREEN_1_get_config_info.vi"("error_in"=w239, "current_time_in"=w237, "reference_name_in"=w238) -> ("error_out"=w233:errorcluster, "current_time_out"=w231:string, "reference_name_out"=w232:string)  [unwired: 6 in]
        n114 = call "OEE_SCREEN_1_get_cycle_time_and_pace.vi"("error_in"=w233, "current_time_in"=w231, "reference_name_in"=w232) -> ("error_out"=w215:errorcluster, "current_time_out"=w216:string, "reference_name_out"=w217:string)  [unwired: 6 in]
        n115 = call "OEE_SCREEN_1_get_availability.vi"("error_in"=w215, "current_time_in"=w216, "reference_name_in"=w217) -> ("error_out"=w230:errorcluster, "current_time_out"=w228:string, "reference_name_out"=w229:string)  [unwired: 6 in]
        n116 = call "OEE_SCREEN_1_get_hourly_ok_count.vi"("error_in"=w230, "current_time_in"=w228, "reference_name_in"=w229) -> ("error_out"=w226:errorcluster)  [unwired: 6 in, 2 out]
        n117 = call "OEE_calculate_targets.vi"("error_in"=w226) -> ("error_out"=w225:errorcluster)  [unwired: 10 in]
        n118 = call "FGV_OEE_SQL_raw_data.vi"("options"=FGV_OEE_SQL_raw_data."get_all_info", "error_in"=w225) -> ("error_out"=w236:errorcluster, "SQL_raw_data_out"=→"SQL_raw_data_out":T1)  [unwired: 8 in]
        n119 = call "OEE_MAIN_check_for_error.vi"("MAIN_loop_state_in"=OEE_MAIN_sequence_state."update_displays", "error_in"=w236) -> ("MAIN_loop_state_out"=w245:T9, "error_out"=w246:errorcluster)  [unwired: 8 in]
      }
      frame "update_displays" {
        n120 = call "OEE_SCREEN_1_update.vi"("error_in"=w265) -> ("error_out"=w264:errorcluster, "SCREEN_1"=w263:T20)  [unwired: 9 in]
        n121 = call "OEE_SCREEN_2_update.vi"("error_in"=w264, "SCREEN_1"=w263) -> ("error_out"=w261:errorcluster, "SCREEN_2"=w249:T21, "SCREEN_1"=w253:T20)  [unwired: 7 in]
        n122 = Unbundle By Name(w262) -> ("queue_refnums.SCREEN_2_queue"=w259:refnum<queue>, "queue_refnums.SCREEN_1_queue"=w260:refnum<queue>)
        n123 = To Variant(anything=w253) -> (Variant=w254:variant)
        n124 = Bundle By Name(cluster=T15 {"state"=enum."update", "variable"=variant} ("element"), "variable"=w254) -> (w255:T15)
        n125 = Enqueue Element(queue=w260, element=w255, error in (no error)=w261) -> (error out=w258:errorcluster)  [unwired: 1 in, 2 out]
        n126 = To Variant(anything=w249) -> (Variant=w252:variant)
        n127 = Bundle By Name(cluster=T17 {"state"=enum."update", "variable"=variant} ("element"), "variable"=w252) -> (w251:T17)
        n128 = Enqueue Element(queue=w259, element=w251, error in (no error)=w258) -> (error out=w257:errorcluster)  [unwired: 1 in, 2 out]
        n129 = call "OEE_MAIN_check_for_error.vi"("MAIN_loop_state_in"=OEE_MAIN_sequence_state."get_next_state", "error_in"=w257) -> ("MAIN_loop_state_out"=w267:T9, "error_out"=w268:errorcluster)  [unwired: 8 in]
      }
      frame "error" {
        n130 = call "FGV_OEE_SQL_connection.vi"("options"=FGV_OEE_SQL_connection."connection_active?", "error_in"=w269) -> ("error_out"=w275:errorcluster, "connection_active?"=w274:bool)  [unwired: 5 in, 3 out]
        n131 = case shown="False" w274 {
          tunnel: [w281 OEE_MAIN_sequence_state."get_next_state" ("OEE_MAIN_sequence_state")] -> w271
          tunnel: [w279 w291] -> w272
          tunnel: w275 -> [w284 w291]
          tunnel: w270 -> [w277 _]
          frame False {
            # "ERROR WITH CONNECTION"
            n132 = Unbundle By Name(w277) -> ("queue_refnums.MAIN_queue"=w276:refnum<queue>)
            n133 = local write "SQL_connection_status"(TRUE ("SQL_connections_indicator_global")) -> ()
            n134 = call "FGV_OEE_SQL_connection.vi"("options"=FGV_OEE_SQL_connection."disconnect", "error_in"=w284) -> ("error_out"=w287:errorcluster)  [unwired: 5 in, 4 out]
            n135 = call <vilib>:"Clear Errors.vi"("error in (no error)"=w287) -> ("error out"=w280:errorcluster)  [unwired: 5 in, 1 out]
            n136 = Preview Queue Element(queue=w276, timeout in ms (-1)=0, error in (no error)=w280) -> (element=w283:T14, error out=w279:errorcluster)  [unwired: 2 out]
            n137 = Unbundle By Name(w283) -> ("state"=w278:T9)
            n138 = case shown="Default" w278 {
              selector: w278 -> [_ w289]
              tunnel: [OEE_MAIN_sequence_state."initialize" ("OEE_MAIN_sequence_state") w289] -> w281
              frame Default {
              }
              frame "stop" {
              }
            }
          }
          frame True {
            # "ERROR WITH SQL STATEMENT OR SIMILAR"
          }
        }
        n139 = call "wait_on_initialization.vi"("state"=w271) -> ()  [unwired: 11 in]
      }
      frame "stop" {
      }
    }
  }
  n140 = while {
    tunnel: w1 -> [w304]
    shift-right: [w301] -> _
    shift-left: w25 -> [w303]
    shift-right: [w300] -> w24
    shift-left: w11 -> [w302]
    shift-right: [w299] -> _
    shift-left: FALSE -> [w298]
    shift-right: [w296] -> _
    shift-left: timestamp(0 s since 1904-01-01) ("current time") -> [w295]
    stop <- w297 stop-if-true
    # "UPDATE PULSE GENERATOR"
    n141 = case shown="\"error\"" w303 {
      tunnel: w304 -> [_ w324 _ _ w348 w362 _]
      tunnel: w302 -> [w310 w323 w332 w338 w350 w357 w370]
      tunnel: [w308 w317 w335 w341 w354 w360 OEE_PULSE_sequence_state."stop" ("OEE_PULSE_sequence_state")] -> w301
      tunnel: [w309 w318 w336 w342 w355 w361 w370] -> w300
      tunnel: [FALSE w322 TRUE FALSE w351 FALSE FALSE] -> w299
      tunnel: w298 -> [_ w322 _ _ w351 _ _]
      tunnel: [_ _ _ _ _ _ TRUE] -> w297
      tunnel: [timestamp(0 s since 1904-01-01) ("current time") w312 w333 w339 w352 w358 w369] -> w296
      tunnel: w295 -> [_ w312 w333 w339 _ w358 w369]
      frame "initialize" {
        n142 = call "OEE_PULSE_check_for_error.vi"("OEE_PULSE_loop_state_in"=OEE_PULSE_sequence_state."get_next_state" ("GUI_TIMER_loop_state_in"), "error_in"=w310) -> ("OEE_PULSE_loop_state_out"=w308:T10, "error_out"=w309:errorcluster)  [unwired: 8 in]
      }
      frame "get_next_state" {
        n143 = Unbundle By Name(w324) -> ("queue_refnums.PULSE_queue"=w325:refnum<queue>, "main_ini_file.Update pulse[ms]"=w311:i32)
        n144 = Select(t=w311, s=w322, f=-1 ("timeout in ms (-1)")) -> (s? t:f=w320:i32)
        n145 = Dequeue Element(queue=w325, timeout in ms (-1)=w320, error in (no error)=w323) -> (element=w315:T13, timed out?=w319:bool, error out=w316:errorcluster)  [unwired: 1 out]
        n146 = case shown="True" w319 {
          tunnel: w316 -> [w328 w331]
          tunnel: w315 -> [w327 _]
          tunnel: [w328 w331] -> w314
          tunnel: [w326 w330] -> w313
          tunnel: w312 -> [_ w329]
          frame False {
            n147 = Unbundle By Name(w327) -> ("state"=w326:T10)
          }
          frame True {
            n148 = call "OEE_PULSE_is_it_time_for_next_pulse.vi"("last_pulse"=w329) -> ("next_state"=w330:T10)  [unwired: 10 in]
          }
        }
        n149 = call "OEE_PULSE_check_for_error.vi"("OEE_PULSE_loop_state_in"=w313, "error_in"=w314) -> ("OEE_PULSE_loop_state_out"=w317:T10, "error_out"=w318:errorcluster)  [unwired: 8 in]
      }
      frame "start_pulses" {
        n150 = call "OEE_PULSE_check_for_error.vi"("OEE_PULSE_loop_state_in"=OEE_PULSE_sequence_state."pulse" ("GUI_TIMER_loop_state_in"), "error_in"=w332) -> ("OEE_PULSE_loop_state_out"=w335:T10, "error_out"=w336:errorcluster)  [unwired: 8 in]
      }
      frame "stop_pulses" {
        n151 = call "OEE_PULSE_check_for_error.vi"("OEE_PULSE_loop_state_in"=OEE_PULSE_sequence_state."get_next_state" ("GUI_TIMER_loop_state_in"), "error_in"=w338) -> ("OEE_PULSE_loop_state_out"=w341:T10, "error_out"=w342:errorcluster)  [unwired: 8 in]
      }
      frame "pulse" {
        n152 = Unbundle By Name(w348) -> ("queue_refnums.MAIN_queue"=w347:refnum<queue>)
        n153 = Enqueue Element(queue=w347, element=T14 {"state"=enum."get_SQL_data", "variable"=variant}, error in (no error)=w350) -> (error out=w349:errorcluster)  [unwired: 1 in, 2 out]
        n154 = local read "update_pulse"() -> (w345:bool)
        n155 = Not(x=w345) -> (.not. x?=w344:bool)
        n156 = local write "update_pulse"(w344) -> ()
        n157 = call "OEE_PULSE_check_for_error.vi"("OEE_PULSE_loop_state_in"=OEE_PULSE_sequence_state."get_next_state" ("GUI_TIMER_loop_state_in"), "error_in"=w349) -> ("OEE_PULSE_loop_state_out"=w354:T10, "error_out"=w355:errorcluster)  [unwired: 8 in]
        n158 = Get Date/Time In Seconds() -> (seconds since 1Jan1904=w352:timestamp)
      }
      frame "error" {
        n159 = Unbundle By Name(w362) -> ("queue_refnums.PULSE_queue"=w366:refnum<queue>)
        n160 = call <vilib>:"Clear Errors.vi"("error in (no error)"=w357) -> ("error out"=w356:errorcluster)  [unwired: 5 in, 1 out]
        n161 = Preview Queue Element(queue=w366, timeout in ms (-1)=0, error in (no error)=w356) -> (element=w364:T13, error out=w361:errorcluster)  [unwired: 2 out]
        n162 = Unbundle By Name(w364) -> ("state"=w365:T10)
        n163 = case shown="Default" w365 {
          tunnel: [OEE_PULSE_sequence_state."initialize" ("OEE_PULSE_sequence_state") OEE_PULSE_sequence_state."stop" ("OEE_PULSE_sequence_state")] -> w360
          frame Default {
          }
          frame "stop" {
          }
        }
        n164 = call "wait_on_initialization.vi"("state"=w360) -> ()  [unwired: 11 in]
      }
      frame "stop" {
      }
    }
  }
  n165 = call "OEE_SCREEN_1.vi"("error_in"=w11, "all_config_info"=w1) -> ("error_out"=w40:errorcluster)  [unwired: 9 in]
  n166 = call "OEE_SCREEN_2.vi"("error_in"=w11, "all_config_info"=w1) -> ("error_out"=w39:errorcluster)  [unwired: 9 in]
  n167 = Merge Errors(w40, w39) -> (w35:errorcluster)
  n168 = Merge Errors(w24, w37, w36, w35) -> (w34:errorcluster)
  n169 = call "OEE_destroy_queues.vi"("error_in"=w34, "all_config_info"=w1) -> ("error_out"=w27:errorcluster)  [unwired: 9 in]
  n170 = control-ref of="This VI"() -> (w29:refnum<vi>)
  n171 = call "close_front_panel_in_exe.vi"("error_in"=w27, "vi_reference_in"=w29) -> ("error_out"=w28:errorcluster)  [unwired: 9 in]
  n172 = call <vilib>:"Clear Errors.vi"("error in (no error)"=w28) -> ()  [unwired: 5 in, 2 out]
